vi "usbsystem set Upstream.vi"(7 "port":u8, 8 "error in (no error)":errorcluster, 9 "index":i32, 10 "result":cluster{"value":i32, "error":i32}, 11 "id":u32) -> (0 "error out":errorcluster, 2 "result out":cluster{"value":i32, "error":i32}, 3 "id out":u32)   [LabVIEW 2021, in "BrainStem2_LabVIEW_Library.lvlib"]
doc: "aLIBEXPORT void __stdcall usbsystem_setUpstream ( unsigned int* id, struct Result* result, const int index , const unsigned char port ) ;"
uses:
  BrainStem2_LabVIEW_Library.lvlib
  BrainStem2_LabVIEW.dll
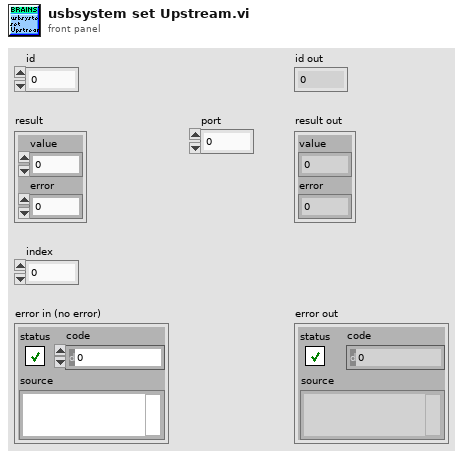
[diagram p1: front panel]
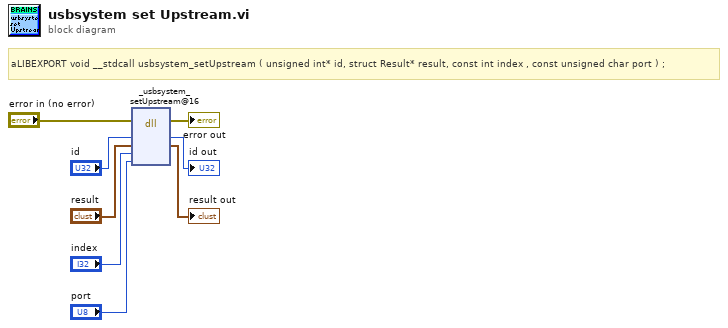
[diagram p0: block diagram]
diagram:
  # "aLIBEXPORT void __stdcall usbsystem_setUpstream ( unsigned int* id, struct Result* result, const int index , const unsigned char port ) ;"
  n1 = dll-call lib="C:/DEV-TDS/Canary/T20029/T20029-80004 BS2 PROG SW/src/drivers/acroname/BrainStem2_LabVIEW.*" fn="_usbsystem_setUpstream@16"(error in="error in (no error)", "id"="id", "result"="result", "index"="index", "port"="port") -> (error out=→"error out":errorcluster, "id"=→"id out":u32, "result"=→"result out":cluster{"value":i32, "error":i32})  [unwired: 5 in, 1 out]
